vi "Connect Core.vi"(4 "queueRef":refnum<queue>, 5 "Commit Only?":bool, 6 "Access (R/W allowed)":T1, 7 "Mode (buffer)":u16(ring)=1 items=["commit", "buffer"], 8 "Error In":errorcluster, 11 "DSCConnection in":refnum<class "DSCConnection.lvclass">) -> (0 "Error Out":errorcluster, 3 "DSCConnection out":refnum<class "DSCConnection.lvclass">)   [LabVIEW 2015, in "CS++DSCConnection.lvlib" / "DSCConnection.lvclass"]
doc: "Open reference to a shared variable if not already connected."
uses:
  DSCConnection.lvclass
  Actors/CS++DSCManager/CS++DSCManager.lvclass
  CSPP_Core/Classes/CS++ProcessVariables/PVConnection/PVConnection.lvclass/PVConnection.ctl
  CSPP_Core/Classes/CS++ProcessVariables/ProcessVariable/PV.lvclass/PV.ctl
  CSPP_Core/Classes/CS++ProcessVariables/ProcessVariable/Read PV URL.vi
  CSPP_Core/Classes/CS++ProcessVariables/ProcessVariable/Read Type Descriptor.vi
  CSPP_Core/Classes/CS++ProcessVariables/ProcessVariable/Read Data.vi
  CSPP_Core/Classes/CS++ProcessVariables/ProcessVariable/PV.lvclass
  CSPP_Core/Classes/CS++ProcessVariables/SVConnection/SVConnection.lvclass
  CSPP_Core/Classes/CS++ProcessVariables/PVConnection/PVConnection.lvclass
  <vilib>/lvdsc/NI_DSC.lvlib
  CSPP_Core/Libraries/Utilities/CS++Utilities.lvlib
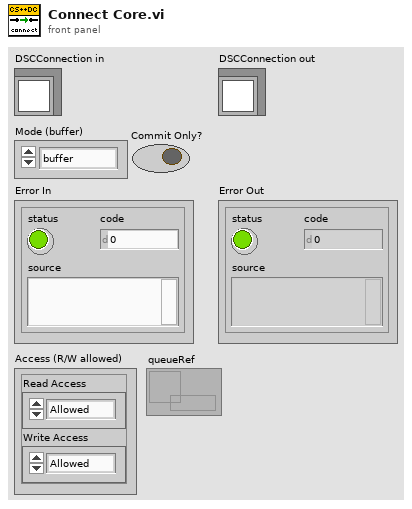
[diagram p1: front panel]
types:
  T1 = cluster{"Read Access":enum8{"Allowed", "Required", "None"}, "Write Access":enum8{"Allowed", "Required", "None"}}
  T2 = enum32{"u32BitField", "bool", "double", "string", "int8", "uint8", "int16", "uint16", "int32", "uint32", "int64", "uint64", "single", "double waveform", "int16 waveform", "array of boolean", "array of int8", "array of uint8", "array of int16", "array of uint16", "array of int32", "array of uint32", "array of int64", "array of uint64", "array of single", "array of double", "array of double waveform", "array of int16 waveform", "array of string", "variant", "timestamp", "fixed point", "custom"}
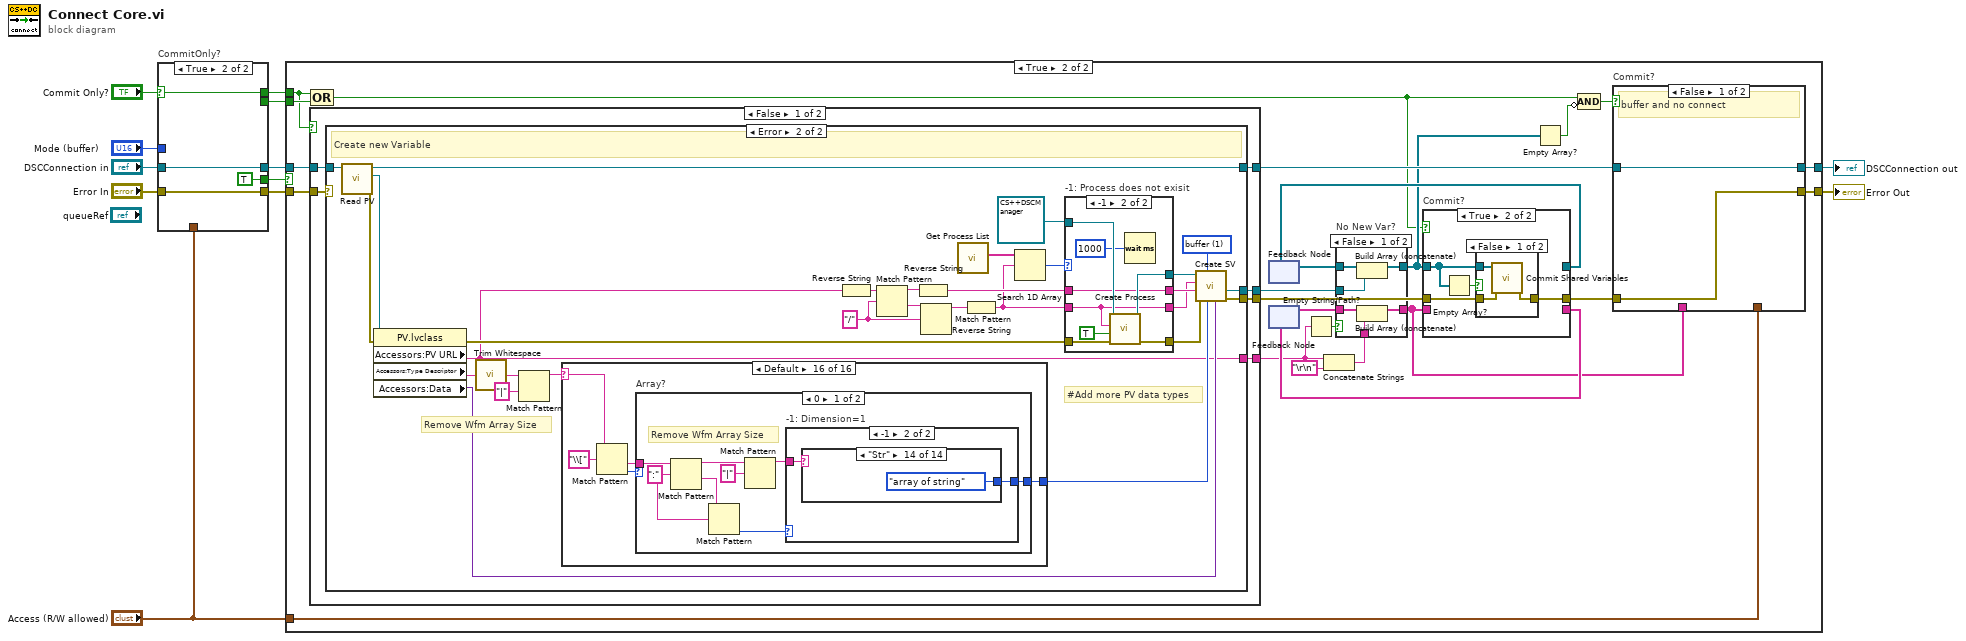
[diagram p0: block diagram]
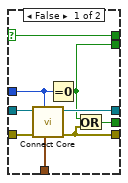
[diagram p2: hidden frame]
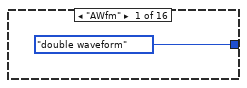
[diagram p6: hidden frame]
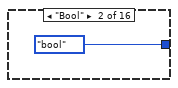
[diagram p7: hidden frame]
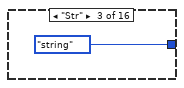
[diagram p8: hidden frame]
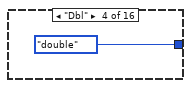
[diagram p9: hidden frame]
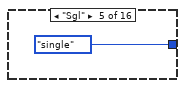
[diagram p10: hidden frame]
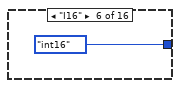
[diagram p11: hidden frame]
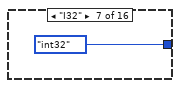
[diagram p12: hidden frame]
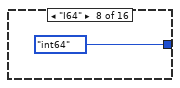
[diagram p13: hidden frame]
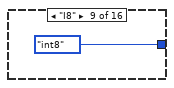
[diagram p14: hidden frame]
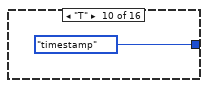
[diagram p15: hidden frame]
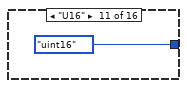
[diagram p16: hidden frame]
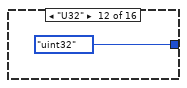
[diagram p17: hidden frame]
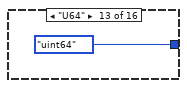
[diagram p18: hidden frame]
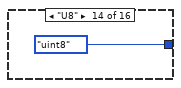
[diagram p19: hidden frame]
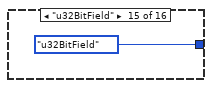
[diagram p20: hidden frame]
diagram:
  n1 = case "CommitOnly?" shown="True" "Commit Only?" {
    selector: "Commit Only?" -> [w13 w25]
    tunnel: "Error In" -> [w21 w22]
    tunnel: "DSCConnection in" -> [w20 w24]
    tunnel: [w19 w24] -> w10
    tunnel: "Access (R/W allowed)" -> [w18 _]
    tunnel: "Mode (buffer)" -> [w17 _]
    tunnel: [w16 TRUE] -> w5
    tunnel: [w15 w22] -> w4
    tunnel: [w14 _] -> w3
    tunnel: [w13 w25] -> w1
    frame False {
      n2 = call-parent "Connect Core.vi"("Access (R/W allowed)"=w18, "Mode (buffer)"=w17, "Error In"=w21, "SVConnection in"=w20) -> ("Error Out"=w15:errorcluster, "SVConnection out"=w19:refnum<class "DSCConnection.lvclass">)  [unwired: 6 in]
      n3 = Equal To 0?(x=w17) -> (x = 0?=w14:bool)
      n4 = Or(x=w14, y=w15) -> (x .or. y?=w16:bool)
    }
    frame True {
    }
  }
  n5 = case shown="True" w5 {
    tunnel: w10 -> [w27 w51]
    tunnel: [w27 w49] -> w9
    tunnel: [w26 w48] -> w8
    tunnel: "Access (R/W allowed)" -> [_ w47]
    tunnel: w4 -> [w26 w36]
    tunnel: w3 -> [_ w29]
    tunnel: w1 -> [_ w28]
    frame False {
    }
    frame True {
      n6 = case shown="False" w28 {
        tunnel: w51 -> [w57 w147]
        tunnel: [w56 w147] -> w50
        tunnel: [w55 _] -> w45
        tunnel: [w54 _] -> w43
        tunnel: w36 -> [w53 _]
        tunnel: [w52 _] -> w32
        frame False {
          n7 = case shown="Error" w53 {
            selector: w53 -> [w58 _]
            tunnel: w57 -> [w59 w88]
            tunnel: [w59 w67] -> w56
            tunnel: [w58 w66] -> w55
            tunnel: [_ w64] -> w54
            tunnel: [_ w63] -> w52
            frame No Error {
              # "Variable already exists"
            }
            frame Error {
              w65 = u16 1 items=["commit", "buffer"] ("Mode (commit)")
              w72 = "/" ("regular expression")
              # "Remove Wfm Array Size"
              # "#Add more PV data types"
              # "Create new Variable"
              n8 = call "Read PV.vi"("PVConnection in"=w88) -> ("error out"=w86:errorcluster, "PV"=w87:refnum<class "PV.lvclass">, "PVConnection out"=w67:refnum<class "DSCConnection.lvclass">)  [unwired: 8 in]
              n9 = property class="PV.lvclass"(reference=w87, error in=w86) -> (error out=w74:errorcluster, "Accessors:PV URL"=w63:string, "Accessors:Type Descriptor"=w83:string, "Accessors:Data"=w81:variant)  [unwired: 1 out]
              n10 = call <vilib>:"Trim Whitespace.vi"("string"=w83) -> ("trimmed string"=w61:string)  [unwired: 1 in]
              n11 = Match Pattern(string=w61, regular expression="|") -> (before substring=w62:string)  [unwired: 1 in, 3 out]
              n12 = case shown="Default" w62 {
                selector: w62 -> [_ _ _ _ _ _ _ _ _ _ _ _ _ _ _ w119]
                tunnel: [T2."double waveform" ("data type") T2."bool" ("data type") T2."string" ("data type") T2."double" ("data type") T2."single" ("data type") T2."int16" ("data type") T2."int32" ("data type") T2."int64" ("data type") T2."int8" ("data type") T2."timestamp" ("data type") T2."uint16" ("data type") T2."uint32" ("data type") T2."uint64" ("data type") T2."uint8" ("data type") T2."u32BitField" ("data type") w120] -> w82
                frame "AWfm" {
                }
                frame "Bool" {
                }
                frame "Str" {
                }
                frame "Dbl" {
                }
                frame "Sgl" {
                }
                frame "I16" {
                }
                frame "I32" {
                }
                frame "I64" {
                }
                frame "I8" {
                }
                frame "T" {
                }
                frame "U16" {
                }
                frame "U32" {
                }
                frame "U64" {
                }
                frame "U8" {
                }
                frame "u32BitField" {
                }
                frame Default {
                  n13 = Match Pattern(string=w119, regular expression="\\[") -> (after substring=w116:string, offset past match=w117:i32)  [unwired: 1 in, 2 out]
                  n14 = case "Array?" shown="0" w117 {
                    tunnel: [w128 T2."variant" ("data type")] -> w120
                    tunnel: w116 -> [w127 _]
                    frame 0 {
                      w125 = ":" ("regular expression")
                      # "Remove Wfm Array Size"
                      n15 = Match Pattern(string=w127, regular expression=w125) -> (before substring=w123:string, after substring=w126:string)  [unwired: 1 in, 2 out]
                      n16 = Match Pattern(string=w126, regular expression=w125) -> (offset past match=w124:i32)  [unwired: 1 in, 3 out]
                      n17 = Match Pattern(string=w123, regular expression="|") -> (before substring=w122:string)  [unwired: 1 in, 3 out]
                      n18 = case "-1: Dimension=1" shown="-1" w124 {
                        tunnel: [T2."variant" ("data type") w131] -> w128
                        tunnel: w122 -> [_ w130]
                        frame Default {
                        }
                        frame -1 {
                          n19 = case shown="\"Str\"" w130 {
                            tunnel: [T2."variant" ("data type") T2."array of boolean" ("data type") T2."array of int8" ("data type") T2."array of uint8" ("data type") T2."array of int16" ("data type") T2."array of uint16" ("data type") T2."array of int32" ("data type") T2."array of uint32" ("data type") T2."array of int64" ("data type") T2."array of uint64" ("data type") T2."array of single" ("data type") T2."array of double" ("data type") T2."array of double waveform" ("data type") T2."array of string" ("data type")] -> w131
                            frame Default {
                            }
                            frame "Bool" {
                            }
                            frame "I8" {
                            }
                            frame "U8" {
                            }
                            frame "I16" {
                            }
                            frame "U16" {
                            }
                            frame "I32" {
                            }
                            frame "U32" {
                            }
                            frame "I64" {
                            }
                            frame "U64" {
                            }
                            frame "Sgl" {
                            }
                            frame "Dbl" {
                            }
                            frame "AWfm" {
                            }
                            frame "Str" {
                            }
                          }
                        }
                      }
                    }
                    frame -1, Default {
                    }
                  }
                }
              }
              n20 = Reverse String(1:w63) -> (0:w85:string)
              n21 = Match Pattern(string=w85, regular expression=w72) -> (before substring=w84:string, after substring=w71:string)  [unwired: 1 in, 2 out]
              n22 = Reverse String(1:w84) -> (0:w76:string)
              n23 = Match Pattern(string=w71, regular expression=w72) -> (before substring=w69:string)  [unwired: 1 in, 3 out]
              n24 = call <vilib>:"Get Process List.vi"() -> ("processes"=w80:string[])  [unwired: 10 in, 1 out]
              n25 = Reverse String(1:w69) -> (0:w68:string)
              n26 = Search 1D Array(1D array=w80, element=w68) -> (index of element=w79:i32)  [unwired: 1 in]
              n27 = case "-1: Process does not exisit" shown="-1" w79 {
                tunnel: [w92 w99] -> w78
                tunnel: refnum<class "CS++DSCManager.lvclass"> refnum ("CS++DSCManager.lvlib:CS++DSCManager.lvclass") -> [w92 w100]
                tunnel: w76 -> [w91 w98]
                tunnel: [w91 w98] -> w75
                tunnel: w74 -> [w90 w97]
                tunnel: [w90 w96] -> w73
                tunnel: w68 -> [w89 w94]
                tunnel: [w89 w94] -> w70
                frame Default {
                }
                frame -1 {
                  n28 = call "Create Process.vi"("Error In"=w97, "Run?"=TRUE, "Process Name"=w94, "CS++DSCManager in"=w100) -> ("Error Out"=w96:errorcluster, "CS++DSCManager out"=w99:refnum<class "CS++DSCManager.lvclass">)  [unwired: 6 in]
                  n29 = Wait (ms)(milliseconds to wait=u32 1000) -> ()  [unwired: 1 out]
                }
              }
              n30 = call "Create SV.vi"("custom control"=w81, "data type"=w82, "Mode (commit)"=w65, "Error In"=w73, "shared variable name"=w75, "process name"=w70, "CS++DSCManager in"=w78) -> ("Error Out"=w66:errorcluster, "Shared Variable"=w64:refnum<k21>)  [unwired: 2 in, 1 out]
            }
          }
        }
        frame True {
        }
      }
      n31 = Compound Arithmetic op=OR(w28, w29) -> (w30:bool)
      n32 = feedback #1() -> (w37:refnum<k21>[])  [unwired: 1 in]
      n33 = feedback #2() -> (w42:string[])  [unwired: 1 in]
      n34 = Empty String/Path?(string/path=w32) -> (empty?=w31:bool)
      n35 = Concatenate Strings(w32, "\r\n") -> (w40:string)
      n36 = case "No New Var?" shown="False" w31 {
        tunnel: w43 -> [w153 _]
        tunnel: w42 -> [w152 w154]
        tunnel: w40 -> [w151 _]
        tunnel: [w150 w154] -> w38
        tunnel: w37 -> [w149 w155]
        tunnel: [w148 w155] -> w35
        frame False {
          n37 = Build Array (concatenate)(w149, w153) -> (w148:refnum<k21>[])
          n38 = Build Array (concatenate)(w152, w151) -> (w150:string[])
        }
        frame True {
        }
      }
      n39 = case "Commit?" shown="True" w30 {
        tunnel: w35 -> [w157 w159]
        tunnel: [w157 _] -> w46
        tunnel: w45 -> [w158 w162]
        tunnel: [w158 w161] -> w44
        tunnel: w38 -> [w156 _]
        tunnel: [w156 _] -> w41
        frame False {
        }
        frame True {
          n40 = Empty Array?(array=w159) -> (empty?=w160:bool)
          n41 = case shown="False" w160 {
            tunnel: w159 -> [w165 _]
            tunnel: w162 -> [w164 w166]
            tunnel: [w163 w166] -> w161
            frame False {
              n42 = call <vilib>:"Commit Shared Variables.vi"("error in (no error)"=w164, "shared variables"=w165) -> ("error out"=w163:errorcluster)  [unwired: 8 in, 1 out]
            }
            frame True {
            }
          }
        }
      }
      n43 = feedback-in #1(w46) -> ()
      n44 = feedback-in #2(w41) -> ()
      n45 = Empty Array?(array=w35) -> (empty?=w34:bool)
      n46 = Compound Arithmetic op=AND(w30, invert w34) -> (w33:bool)
      n47 = case "Commit?" shown="False" w33 {
        tunnel: w44 -> [w167 w173]
        tunnel: w50 -> [w168 w175]
        tunnel: [w168 w174] -> w49
        tunnel: [w167 w172] -> w48
        tunnel: w47 -> [_ w171]
        tunnel: w38 -> [_ w169]
        frame False {
          # "buffer and no connect"
        }
        frame True {
          # "commit & connect"
          n48 = flat-sequence {
            tunnel: w175 -> [w181]
            tunnel: [w181] -> w170
            tunnel: w169 -> [w176]
            tunnel: [w185] -> w174
            tunnel: w173 -> [w184]
            tunnel: [w183] -> w172
            tunnel: w171 -> [w182]
            tunnel: w170 -> [w186]
            frame #0 {
              n49 = Concatenate Strings("Deploying SV...", "\r\n", w176) -> (w178:string)
              n50 = call "Floating Messagebox.vi"("Timeout"=dbl[unit] 60.0, "Display Message"=w178) -> ()  [unwired: 1 in, 1 out]
            }
            frame #1 {
              n51 = call-parent "Connect Core.vi"("Access (R/W allowed)"=w182, "Error In"=w184, "SVConnection in"=w186) -> ("Error Out"=w183:errorcluster, "SVConnection out"=w185:refnum<class "DSCConnection.lvclass">)  [unwired: 7 in]
            }
          }
        }
      }
    }
  }
  "Error Out" <- w8
  "DSCConnection out" <- w9
